vi "File loader.vi"(0 "File style in":u16(ring) items=["Sequential files", "Single database"], 1 "Files in":path[](array[path]), 2 "File number to display":i32, 3 "Xcol":i16, 4 "Ycol":i16, 5 "Delim":string) -> (14 "File name":string, 15 "Xdata":dbl[](array[numeric]), 18 "Ydata":dbl[](array[numeric]))   [LabVIEW 2014]
uses:
  <vilib>/Utility/file.llb/Read From Spreadsheet File (DBL).vi
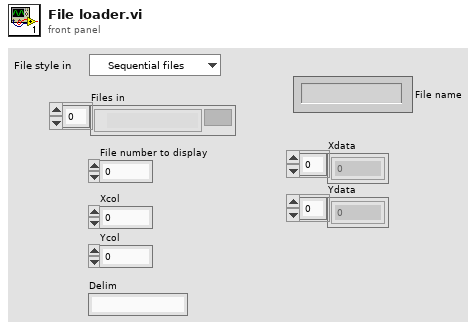
[diagram p1: front panel]
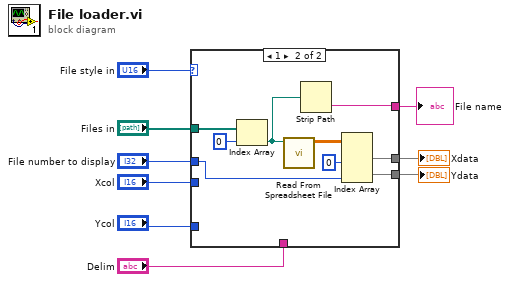
[diagram p0: block diagram]
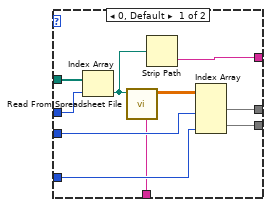
[diagram p2: hidden frame]
diagram:
  n1 = case shown="1" "File style in" {
    tunnel: "File number to display" -> [w19 w22]
    tunnel: "Ycol" -> [w18 _]
    tunnel: "Xcol" -> [w17 _]
    tunnel: "Files in" -> [w15 w28]
    tunnel: "Delim" -> [w14 _]
    tunnel: [w13 w25] -> w4
    tunnel: [w12 w24] -> w3
    tunnel: [w10 w20] -> w1
    frame 0, Default {
      n2 = Index Array(array=w15, index=w19) -> (element=w11:path)
      n3 = call-poly <vilib>:"Read From Spreadsheet File.vi"("delimiter (\\t)"=w14, "file path (dialog if empty)"=w11) -> ("all rows"=w16:dbl[][])  [unwired: 5 in, 4 out]
      n4 = Strip Path(path=w11) -> (name=w10:string)  [unwired: 1 out]
      n5 = Index Array(array=w16, index (col) #1=w17, index (col) #2=w18) -> (element #1=w13:dbl[], element #2=w12:dbl[])  [unwired: 2 in]
    }
    frame 1 {
      n6 = Index Array(array=w28, index=0) -> (element=w21:path)
      n7 = call-poly <vilib>:"Read From Spreadsheet File.vi"("file path (dialog if empty)"=w21) -> ("all rows"=w26:dbl[][])  [unwired: 6 in, 4 out]
      n8 = Strip Path(path=w21) -> (name=w20:string)  [unwired: 1 out]
      n9 = Index Array(array=w26, index (col) #1=0, index (col) #2=w22) -> (element #1=w25:dbl[], element #2=w24:dbl[])  [unwired: 2 in]
    }
  }
  "Xdata" <- w4
  "Ydata" <- w3
  "File name" <- w1
